vi "ReadJigBarcode.vi"() -> (1 "OK":bool, 2 "P":bool, 3 "SmallProduct":bool, 4 "SP":bool)   [LabVIEW 2014]
uses:
  axxon_Gold.vi
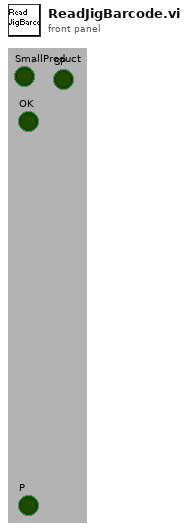
[diagram p1: front panel]
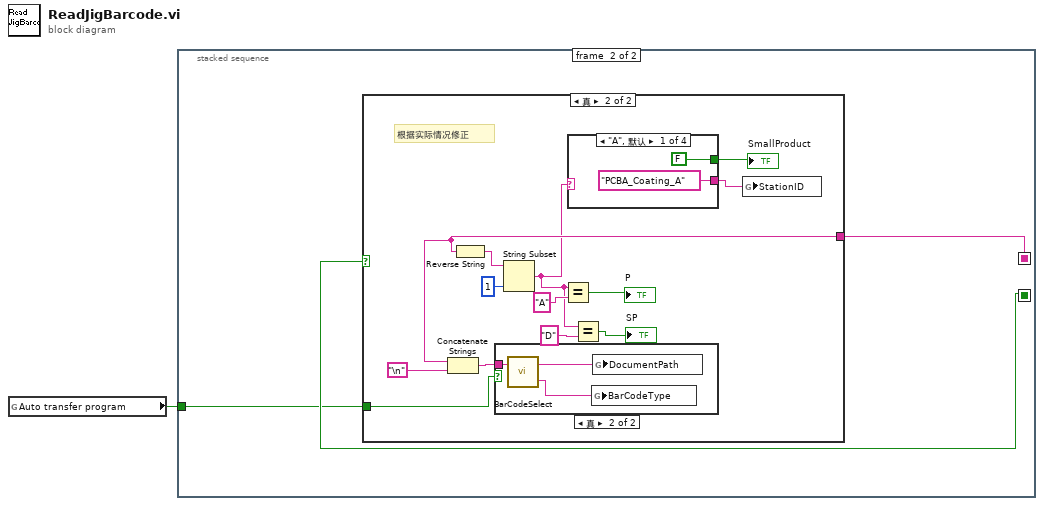
[diagram p0: block diagram]
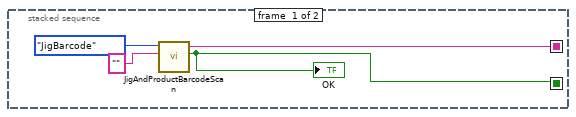
[diagram p2: hidden frame]
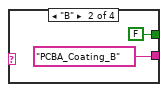
[diagram p5: hidden frame]
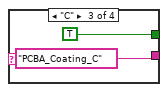
[diagram p6: hidden frame]
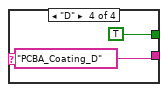
[diagram p7: hidden frame]
diagram:
  n1 = global read "axxon_Gold.vi" "Auto transfer program"() -> (w1:bool)
  n2 = stacked-sequence {
    seq-local: [w3 _] -> [_ w8]
    seq-local: [w5 _] -> [_ w7]
    tunnel: w1 -> [_ w6]
    frame #0 {
      n3 = call "JigAndProductBarcodeScan.vi"("Barcode"="" ("条码"), "BarcodePosition"=enum16{"JigBarcode", "ProductBarcode"}."JigBarcode") -> ("OK"=w5:bool, "条码输出"=w3:string)  [unwired: 8 in]
      "OK" <- w5
    }
    frame #1 {
      n4 = case shown="真" w7 {
        tunnel: w8 -> [_ w21]
        tunnel: w6 -> [_ w9]
        frame False {
        }
        frame True {
          # "根据实际情况修正"
          n5 = Concatenate Strings(w21, "\n") -> (w18:string)
          n6 = Reverse String(1:w21) -> (0:w16:string)
          n7 = case shown="真" w9 {
            tunnel: w18 -> [_ w22]
            frame False {
            }
            frame True {
              n8 = call "BarCodeSelect.vi"("BarcodeIn"=w22) -> ("ProductTyple"=w23:string, "ProgramPath"=w24:string)  [unwired: 1 in]
              n9 = global write "axxon_Gold.vi" "BarCodeType"(w23) -> ()
              n10 = global write "axxon_Gold.vi" "DocumentPath"(w24) -> ()
            }
          }
          n11 = String Subset(string=w16, length (rest)=1 ("长度（剩余）")) -> (substring=w12:string)  [unwired: 1 in]
          n12 = Equal?(x=w12, y="A") -> (x = y?=→"P":bool)
          n13 = case shown="\"A\", 默认" w12 {
            tunnel: ["PCBA_Coating_A" ("y") "PCBA_Coating_B" ("y") "PCBA_Coating_C" ("y") "PCBA_Coating_D" ("y")] -> w15
            tunnel: [FALSE ("小产品") FALSE ("小产品") TRUE ("小产品") TRUE ("小产品")] -> w14
            frame "A", Default {
            }
            frame "B" {
            }
            frame "C" {
            }
            frame "D" {
            }
          }
          "SmallProduct" <- w14
          n14 = Equal?(x=w12, y="D") -> (x = y?=→"SP":bool)
          n15 = global write "axxon_Gold.vi" "StationID"(w15) -> ()
        }
      }
    }
  }
